vi "add_one_control_command.vi"(8 "error in":errorcluster, 9 "Controls Specs":T1[](array[typedef]), 10 "Instrument Command":string, 11 "VI Ref In":refnum<vi>) -> (0 "error out":errorcluster, 3 "VI Ref Out":refnum<vi>)   [LabVIEW 2018]
uses:
  TypeDefinitions/single_control_spec.ctl
  TypeDefinitions/control_data_type.ctl
  TypeDefinitions/control_class.ctl
  TypeDefinitions/ring_string_and_value.ctl
  Iternl/ConverttStr/TypeDefinitions/conver_strings_types.ctl
  Misc/AddNode/TypeDefinitions/node_types.ctl
  Iternl/CalPos/CmdToStr/TypeDefinitions/main_position_types.ctl
  Iternl/GetNodeTerm/StringProcessingNode/TypeDefinitions/string_node_type.ctl
  Iternl/ConttWire/TypeDefines/connect_with_last_node_types.ctl
  Iternl/AddObj/AddControl/TypeDefinitions/bd_control_type.ctl
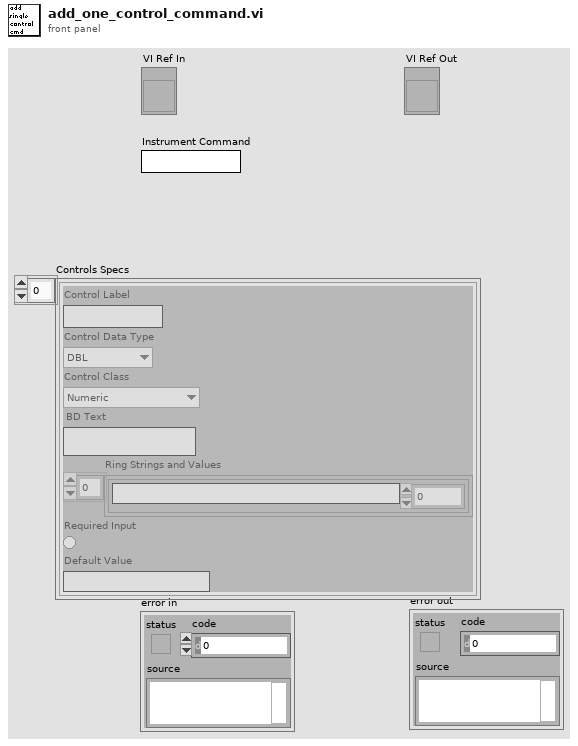
[diagram p1: front panel]
types:
  T1 = typedef "single_control_spec.ctl" = cluster{"Control Label":string, "Control Data Type":T2, "Control Class":T3, "BD Text":string, "Ring Strings and Values":T4[], "Required Input":bool, "Default Value":string}
  T2 = typedef "control_data_type.ctl" = enum16{"DBL", "I32", "Boolean", "String", "U16", "U32", "EXT", "SGL", "I16", "U8", "I8", "I64", "U64", "Waveform", "Reference", "Variant", "Cluster"}
  T3 = typedef "control_class.ctl" = enum16{"Numeric", "Vertical Slide Switch", "Text Ring", "String", "Array", "VISAName", "WaveformGraph", "Cluster"}
  T4 = typedef "ring_string_and_value.ctl" = cluster{"String":string, "Value":dbl}
  T5 = typedef "string_node_type.ctl" = enum16{"FormatIntoString", "PickLine", "AppendTrueFalse", "ConcatenateStrings"}
  T6 = typedef "main_position_types.ctl" = enum16{"Node", "FormatNodeForMultipleControls", "BoolConstant", "FormatConstant", "1stSubNodeX"}
  T7 = typedef "node_types.ctl" = enum16{"FormatIntoString", "PickLine", "AppendTrueFalse", "VISAWrite", "SubVI", "ConcatenateStrings", "VISARead", "ProperyNode", "ScanFromString", "SpreadSheetStringToArray"}
  T8 = typedef "conver_strings_types.ctl" = enum16{"BooleanCMD", "RingCMD"}
  T9 = typedef "bd_control_type.ctl" = enum16{"Numeric", "Ring", "Boolean", "String", "VisaIn", "VisaOut", "Error In", "Error Out", "Array", "Waveform"}
  T10 = typedef "connect_with_last_node_types.ctl" = u16
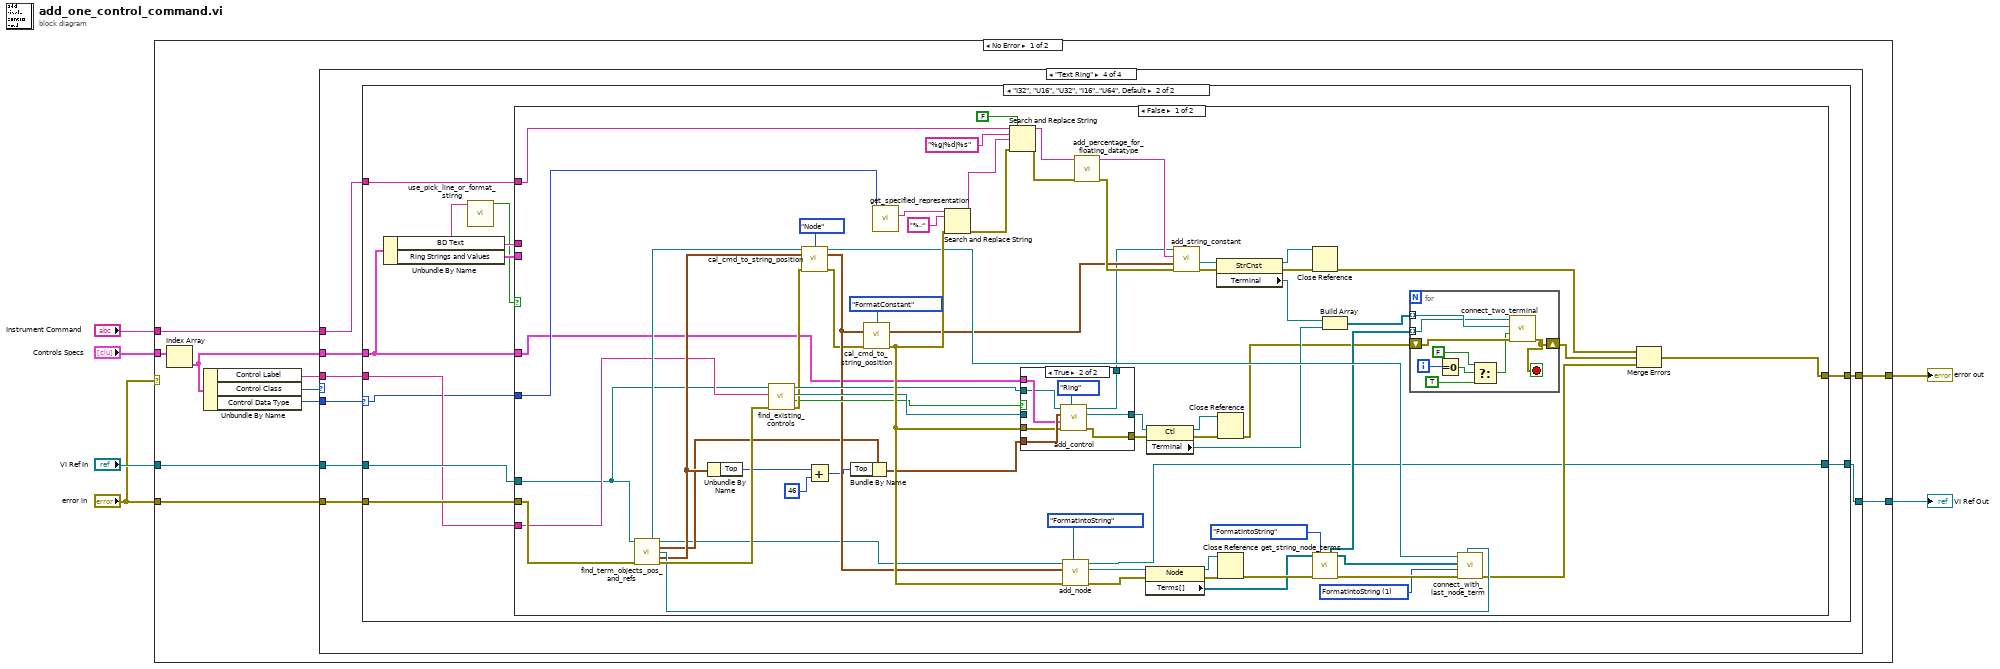
[diagram p0: block diagram]
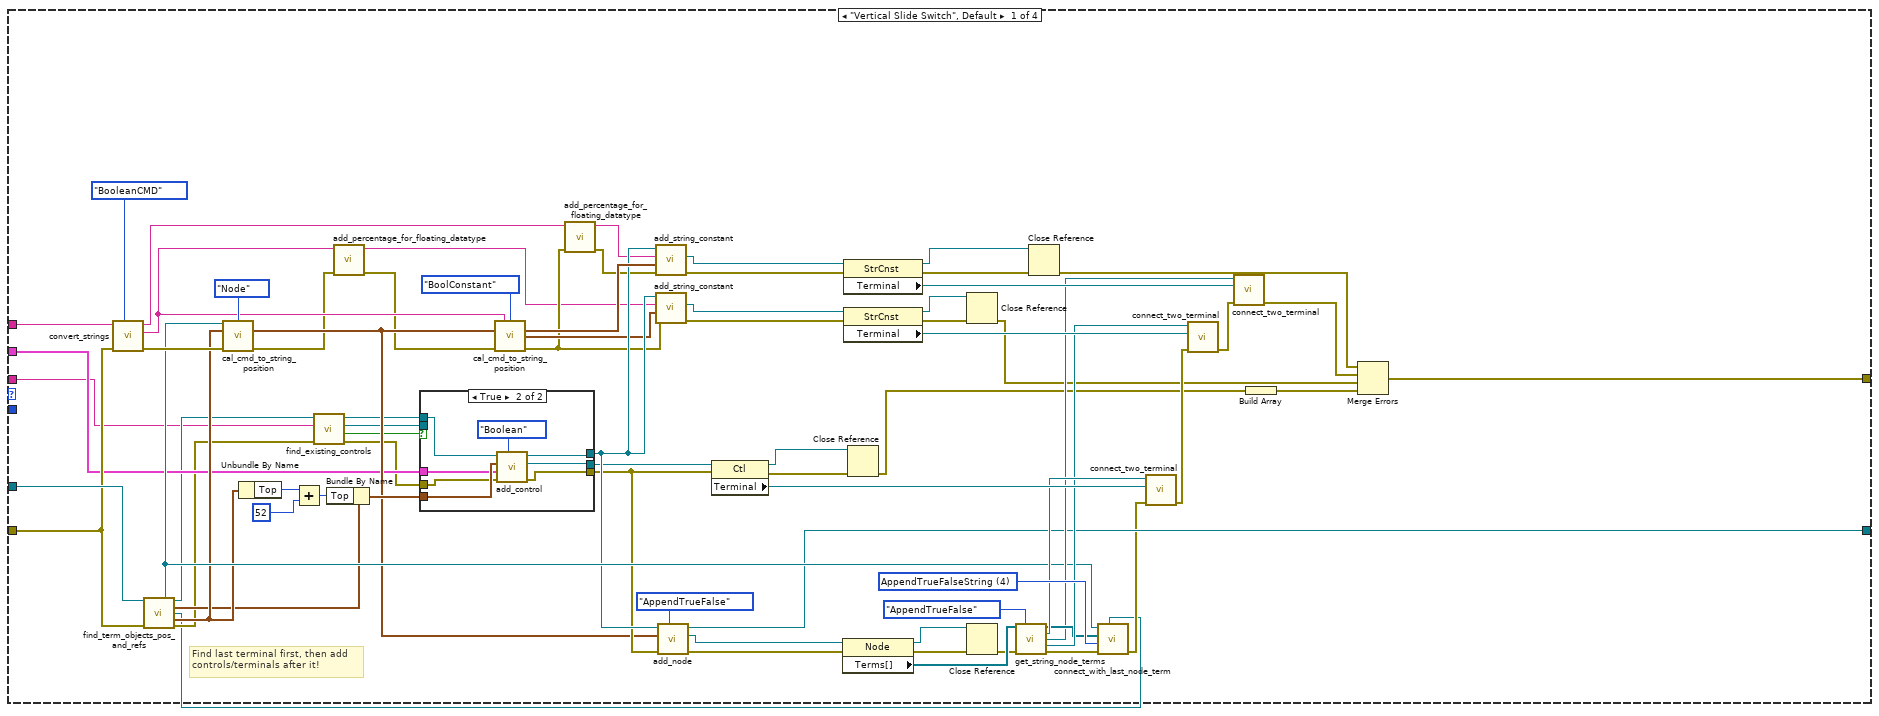
[diagram p2: hidden frame]
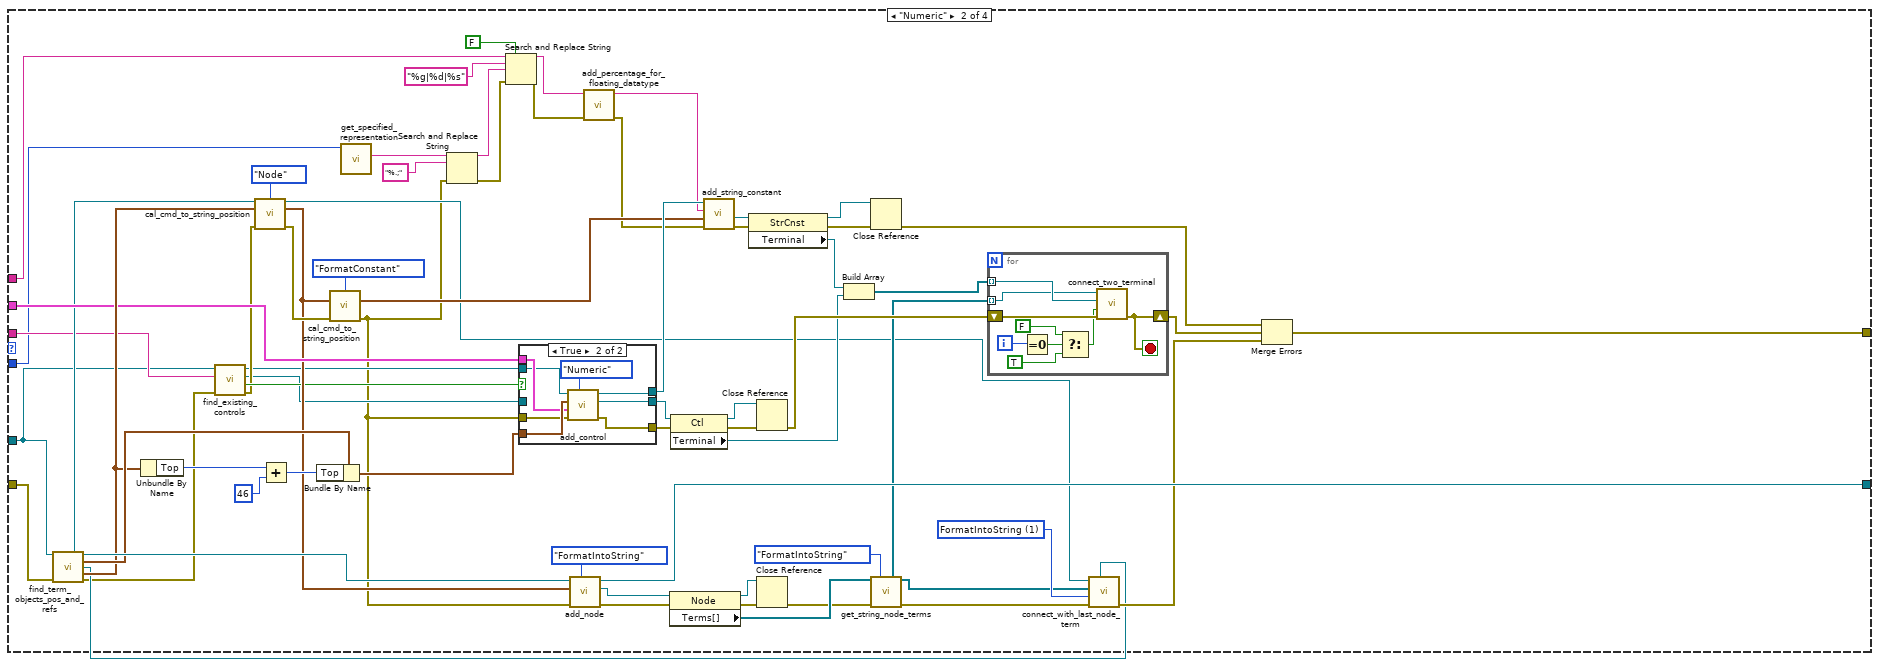
[diagram p4: hidden frame]
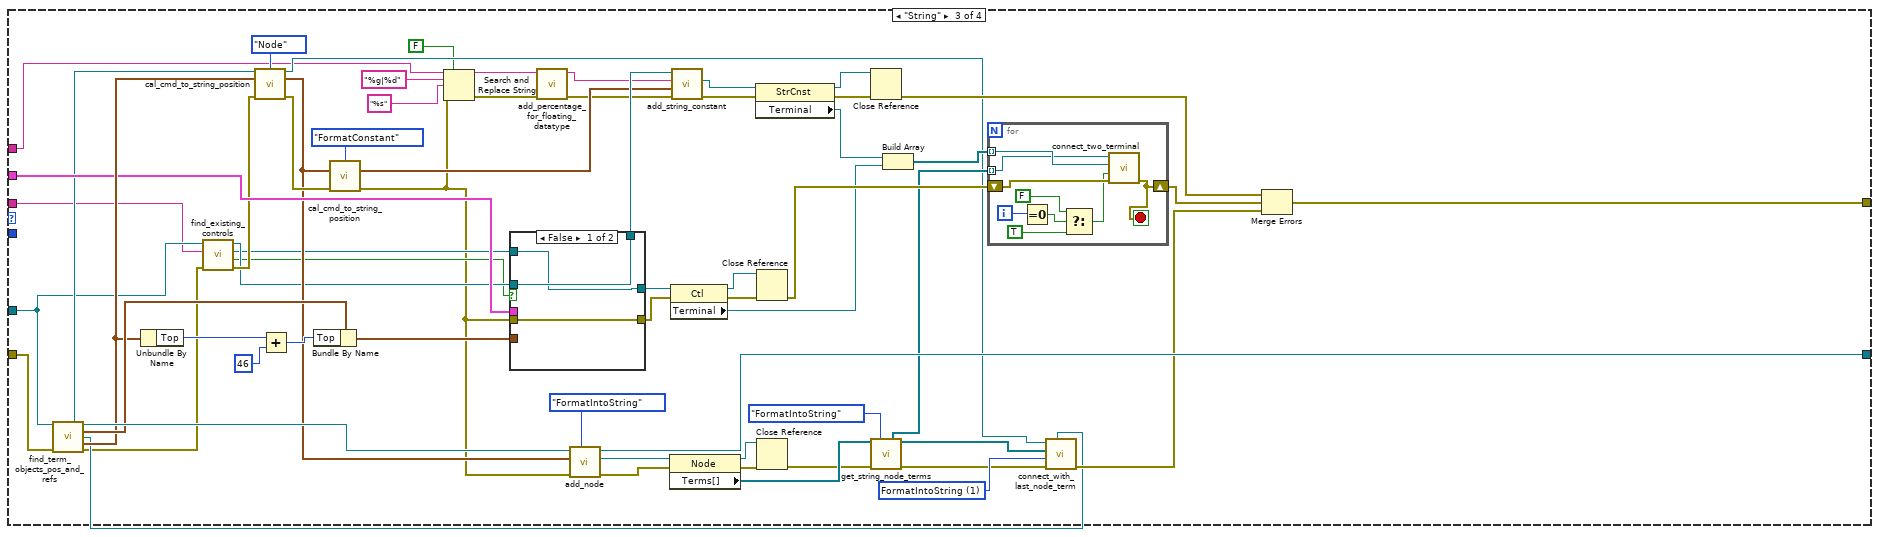
[diagram p6: hidden frame]
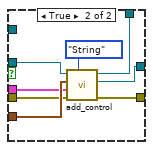
[diagram p7: hidden frame]
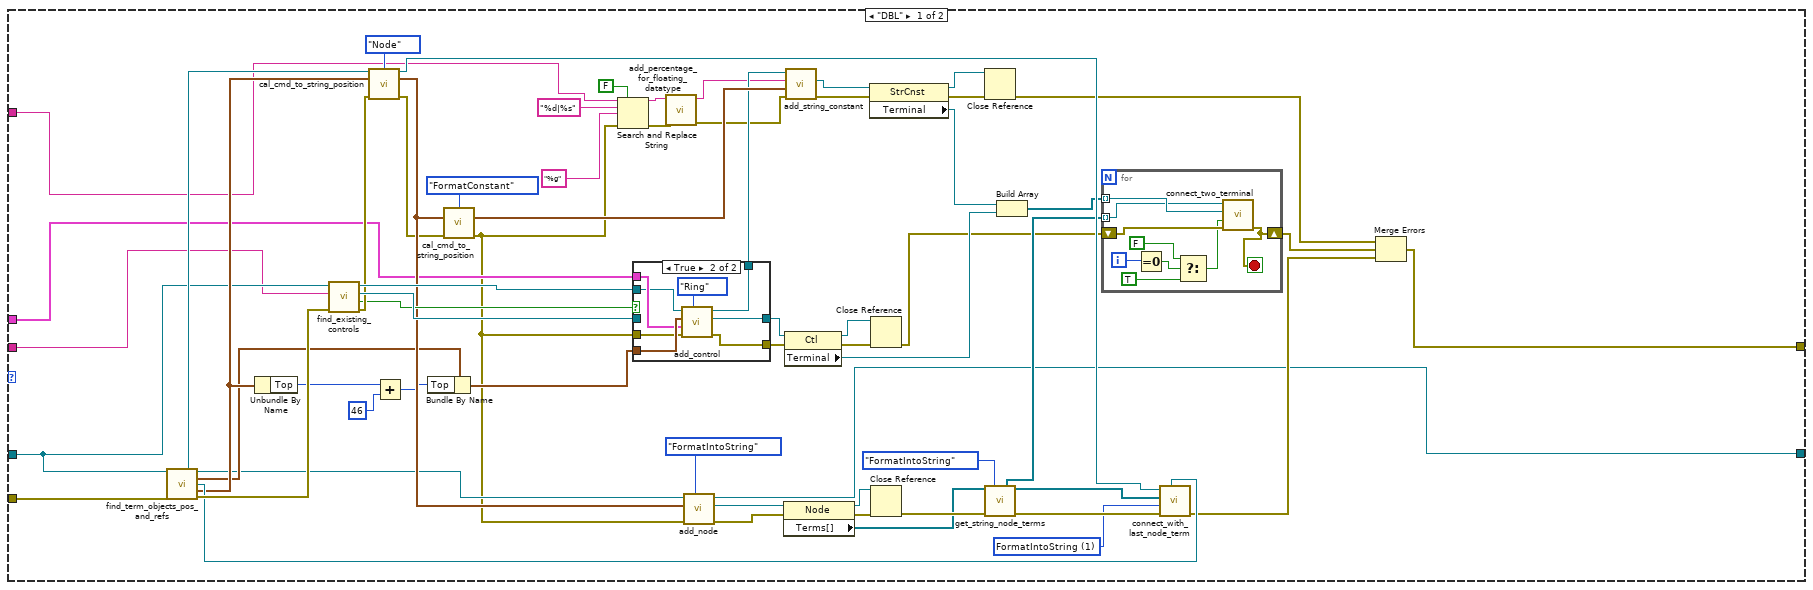
[diagram p8: hidden frame]
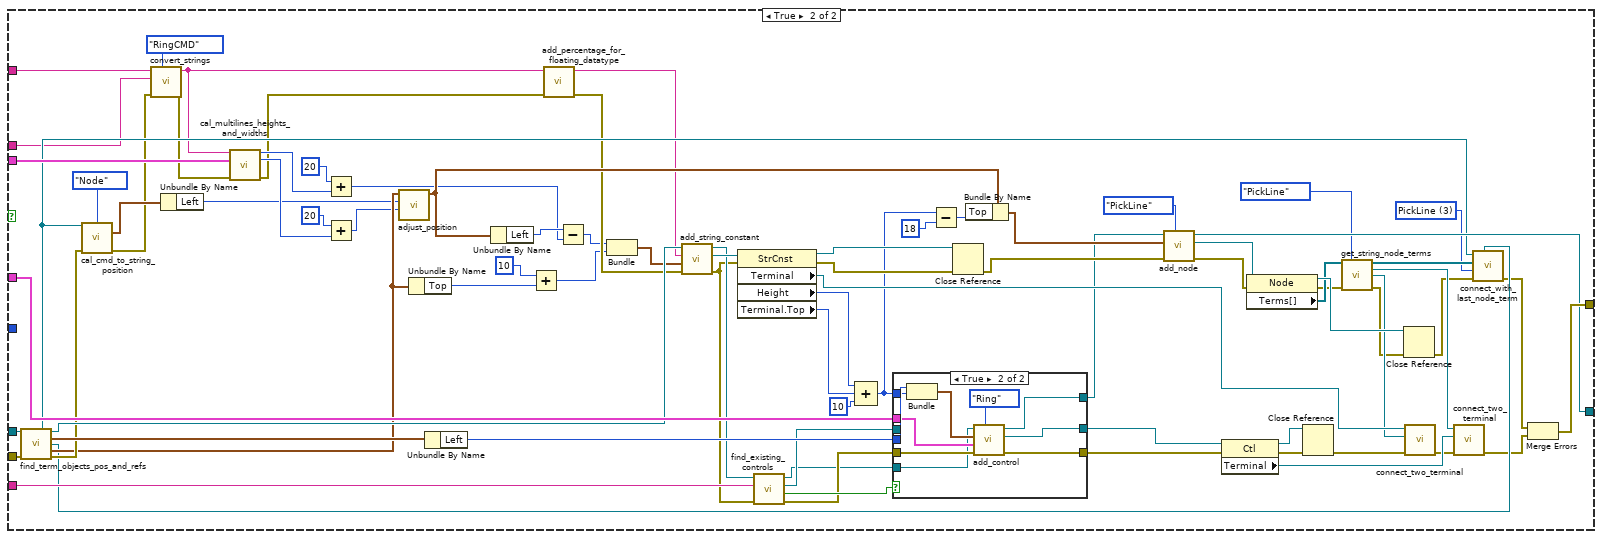
[diagram p11: hidden frame]
diagram:
  n1 = case shown="No Error" "error in" {
    selector: "error in" -> [_ w555]
    tunnel: "error in" -> [w15 _]
    tunnel: [w14 w555] -> w6
    tunnel: "Instrument Command" -> [w13 _]
    tunnel: [w11 w554] -> w4
    tunnel: "VI Ref In" -> [w10 w554]
    tunnel: "Controls Specs" -> [w9 _]
    frame No Error {
      n2 = Index Array(array=w9) -> (element=w16:T1)  [unwired: 1 in]
      n3 = Unbundle By Name(w16) -> ("Control Label"=w8:string, "Control Class"=w12:T3, "Control Data Type"=w7:T2)
      n4 = case shown="\"Text Ring\"" w12 {
        tunnel: w10 -> [w56 w120 w204 w277]
        tunnel: [w52 w154 w237 w275] -> w11
        tunnel: w16 -> [w48 w131 w214 w274]
        tunnel: w13 -> [w90 w113 w197 w279]
        tunnel: [w89 w139 w222 w276] -> w14
        tunnel: w15 -> [w55 w138 w221 w278]
        tunnel: w8 -> [w28 w121 w201 w273]
        tunnel: w7 -> [_ w112 _ w272]
        frame "Vertical Slide Switch", Default {
          w88 = T10 4 items=["AppendTrueFalseString"=4, "PickLine"=3, "FormatIntoString"=1] ("Terminal Index")
          # "Find last terminal first, then add \ncontrols/terminals after it!"
          n5 = call "convert_strings.vi"("Enum"=conver_strings_types."BooleanCMD", "error in (no error)"=w55, "Instrument Command"=w90) -> ("error out"=w86:errorcluster, "Disable String"=w21:string, "Ring CMD/Enable String"=w25:string)  [unwired: 1 in, 5 out]
          n6 = call "find_term_objects_pos_and_refs.vi"("VI Ref In"=w56, "error in (no error)"=w55) -> ("Last Function"=w63:refnum<vi>, "VI Ref Out"=w32:refnum<vi>, "Last Control Position"=w59:cluster{"Left":i32, "Top":i32}, "Last StrCnst Refnum"=w17:refnum<vi>, "Last Function Position"=w60:cluster{"Left":i32, "Top":i32}, "error out"=w31:errorcluster)  [unwired: 8 out]
          n7 = call "cal_cmd_to_string_position.vi"("Last Function Ref In"=w63, "Enum"=main_position_types."Node", "Main Node BD Position"=w60, "error in (no error)"=w86) -> ("Main Node Position/Enable Constant Position"=w49:cluster{"Left":u32, "Top":i32}, "error out"=w20:errorcluster)  [unwired: 3 in, 7 out]
          n8 = Unbundle By Name(w60) -> ("Top"=w58:i32)
          n9 = Add(x=w58, y=52) -> (x+y=w61:i32)
          n10 = call "find_existing_controls.vi"("error in (no error)"=w31, "Label Text"=w28, "VI Ref In"=w32) -> ("error out"=w30:errorcluster, "New Ctrl"=w26:bool, "Ctrl Ref Out"=w27:refnum<vi>, "VI Ref Out"=w29:refnum<vi>)  [unwired: 5 out]
          n11 = Bundle By Name(cluster=w59, "Top"=w61) -> (w57:cluster{"Left":i32, "Top":i32})
          n12 = call "add_percentage_for_floating_datatype.vi"("error in (no error)"=w20, "String In"=w21) -> ("error out"=w19:errorcluster, "String Out"=w18:string)  [unwired: 8 out]
          n13 = case shown="True" w26 {
            tunnel: w57 -> [_ w101]
            tunnel: [w93 w100] -> w54
            tunnel: [w91 w99] -> w50
            tunnel: w48 -> [_ w98]
            tunnel: [w92 w97] -> w44
            tunnel: w30 -> [w91 w95]
            tunnel: w29 -> [w93 w94]
            tunnel: w27 -> [w92 _]
            frame False {
            }
            frame True {
              n14 = call "add_control.vi"("Add Control Type"=bd_control_type."Boolean" ("Enum"), "error in (no error)"=w95, "Single Control Spec"=w98, "BD Position"=w101, "VI Ref In"=w94) -> ("error out"=w99:errorcluster, "Control Ref Out"=w97:refnum<vi>, "VI Ref Out"=w100:refnum<vi>)  [unwired: 4 out]
            }
          }
          n15 = call "cal_cmd_to_string_position.vi"("Disable String"=w21, "Enum"=main_position_types."BoolConstant", "Main Node BD Position"=w49, "error in (no error)"=w19) -> ("Main Node Position/Enable Constant Position"=w87:cluster{"Left":u32, "Top":i32}, "Disable Constant Position"=w36:cluster{u32, i32}, "error out"=w23:errorcluster)  [unwired: 3 in, 6 out]
          n16 = call "add_percentage_for_floating_datatype.vi"("error in (no error)"=w23, "String In"=w25) -> ("error out"=w22:errorcluster, "String Out"=w24:string)  [unwired: 8 out]
          n17 = call "add_string_constant.vi"("error in"=w22, "BD Position"=w87, "StringConstantValue"=w24, "VI Ref In"=w54) -> ("error out"=w84:errorcluster, "StrCnst Refnum"=w83:refnum<vi>)  [unwired: 6 out]
          n18 = call "add_string_constant.vi"("error in"=w23, "BD Position"=w36, "StringConstantValue"=w18, "VI Ref In"=w54) -> ("error out"=w85:errorcluster, "StrCnst Refnum"=w82:refnum<vi>)  [unwired: 6 out]
          n19 = call "add_node.vi"("Node Type"=node_types."AppendTrueFalse", "error in (no error)"=w50, "BD Position"=w49, "VI Ref In"=w54) -> ("error out"=w51:errorcluster, "Node Refnum"=w53:refnum<vi>, "VI Ref Out"=w52:refnum<vi>)  [unwired: 2 in, 3 out]
          n20 = property class="Ctl"(reference=w44, error in=w50) -> (reference out=w75:refnum<vi>, error out=w74:errorcluster, "Terminal"=w81:refnum<vi>)
          n21 = property class="Node"(reference=w53, error in=w51) -> (reference out=w73:refnum<vi>, error out=w72:errorcluster, "Terms[]"=w80:refnum<vi>[])
          n22 = property class="StrCnst"(reference=w83, error in=w84) -> (reference out=w70:refnum<vi>, error out=w69:errorcluster, "Terminal"=w79:refnum<vi>)
          n23 = property class="StrCnst"(reference=w82, error in=w85) -> (reference out=w68:refnum<vi>, error out=w67:errorcluster, "Terminal"=w78:refnum<vi>)
          n24 = Close Reference(reference=w75, error in (no error)=w74) -> (error out=w40:errorcluster)
          n25 = Close Reference(reference=w68, error in (no error)=w67) -> (error out=w41:errorcluster)
          n26 = Close Reference(reference=w73, error in (no error)=w72) -> (error out=w71:errorcluster)
          n27 = call "get_string_node_terms.vi"("Terms[] In"=w80, "Node Type"=string_node_type."AppendTrueFalse", "error in (no error)"=w71) -> ("Terms[]  Out"=w66:refnum<vi>[], "Pick Term"=w77:refnum<vi>, "Multiline Term/Enable Term/Concantenate Term"=w65:refnum<vi>, "Pick Line Output Term/Disable Term"=w76:refnum<vi>, "error out"=w64:errorcluster)  [unwired: 1 in, 7 out]
          n28 = Close Reference(reference=w70, error in (no error)=w69) -> (error out=w46:errorcluster)
          n29 = call "connect_with_last_node_term.vi"("Last StrCnst Refnum"=w17, "error in (no error)"=w64, "Terminal Index"=w88, "Terminals[]"=w66, "Last Function Ref In"=w63) -> ("error out"=w43:errorcluster)  [unwired: 6 out]
          n30 = call "connect_two_terminal.vi"("error in"=w43, "Terminal 2"=w81, "Terminal 1"=w77) -> ("error out"=w42:errorcluster)  [unwired: 1 in, 7 out]
          n31 = call "connect_two_terminal.vi"("error in"=w42, "Terminal 2"=w78, "Terminal 1"=w76) -> ("error out"=w47:errorcluster)  [unwired: 1 in, 7 out]
          n32 = call "connect_two_terminal.vi"("error in"=w47, "Terminal 2"=w79, "Terminal 1"=w65) -> ("error out"=w45:errorcluster)  [unwired: 1 in, 7 out]
          n33 = Build Array(w40) -> (w39:errorcluster[])
          n34 = Merge Errors(w46, w45, w41, w39) -> (w89:errorcluster)
        }
        frame "Numeric" {
          w168 = T10 1 items=["AppendTrueFalseString"=4, "PickLine"=3, "FormatIntoString"=1] ("Terminal Index")
          n35 = call "find_term_objects_pos_and_refs.vi"("VI Ref In"=w120, "error in (no error)"=w138) -> ("Last Function"=w127:refnum<vi>, "VI Ref Out"=w149:refnum<vi>, "Last Control Position"=w136:cluster{"Left":i32, "Top":i32}, "Last StrCnst Refnum"=w122:refnum<vi>, "Last Function Position"=w133:cluster{"Left":i32, "Top":i32}, "error out"=w119:errorcluster)  [unwired: 8 out]
          n36 = Unbundle By Name(w133) -> ("Top"=w132:i32)
          n37 = call "find_existing_controls.vi"("error in (no error)"=w119, "Label Text"=w121, "VI Ref In"=w120) -> ("error out"=w117:errorcluster, "New Ctrl"=w118:bool, "Ctrl Ref Out"=w115:refnum<vi>, "VI Ref Out"=w116:refnum<vi>)  [unwired: 5 out]
          n38 = call "cal_cmd_to_string_position.vi"("Last Function Ref In"=w127, "Enum"=main_position_types."Node", "Main Node BD Position"=w133, "error in (no error)"=w117) -> ("Last Function Ref Out"=w126:refnum<vi>, "Main Node Position/Enable Constant Position"=w129:cluster{"Left":u32, "Top":i32}, "error out"=w167:errorcluster)  [unwired: 3 in, 6 out]
          n39 = Add(x=w132, y=46) -> (x+y=w134:i32)
          n40 = Bundle By Name(cluster=w136, "Top"=w134) -> (w135:cluster{"Left":i32, "Top":i32})
          n41 = call "cal_cmd_to_string_position.vi"("Enum"=main_position_types."FormatConstant", "Main Node BD Position"=w129, "error in (no error)"=w167) -> ("Main Node Position/Enable Constant Position"=w128:cluster{"Left":u32, "Top":i32}, "error out"=w107:errorcluster)  [unwired: 4 in, 7 out]
          n42 = call "get_specified_representation.vi"("Control Data Type"=w112) -> ("Format String"=w110:string)  [unwired: 10 out]
          n43 = Search and Replace String(input string=w110, search string="%.;", error in=w107) -> (result string=w108:string, error out=w106:errorcluster)  [unwired: 7 out]
          n44 = Search and Replace String(replace all?=FALSE ("replace all? (F)"), input string=w113, search string="%g|%d|%s", replace string=w108, error in=w106) -> (result string=w104:string, error out=w103:errorcluster)  [unwired: 5 out]
          n45 = case shown="True" w118 {
            tunnel: [w170 w179] -> w151
            tunnel: [w171 w178] -> w150
            tunnel: [w169 w177] -> w148
            tunnel: w135 -> [_ w176]
            tunnel: w107 -> [w169 w175]
            tunnel: w131 -> [_ w174]
            tunnel: w116 -> [w171 w172]
            tunnel: w115 -> [w170 _]
            frame False {
            }
            frame True {
              n46 = call "add_control.vi"("Add Control Type"=bd_control_type."Numeric" ("Enum"), "error in (no error)"=w175, "Single Control Spec"=w174, "BD Position"=w176, "VI Ref In"=w172) -> ("error out"=w177:errorcluster, "Control Ref Out"=w179:refnum<vi>, "VI Ref Out"=w178:refnum<vi>)  [unwired: 4 out]
            }
          }
          n47 = call "add_node.vi"("Node Type"=node_types."FormatIntoString", "error in (no error)"=w107, "BD Position"=w129, "VI Ref In"=w149) -> ("error out"=w165:errorcluster, "Node Refnum"=w140:refnum<vi>, "VI Ref Out"=w154:refnum<vi>)  [unwired: 2 in, 3 out]
          n48 = call "add_percentage_for_floating_datatype.vi"("error in (no error)"=w103, "String In"=w104) -> ("error out"=w102:errorcluster, "String Out"=w105:string)  [unwired: 8 out]
          n49 = property class="Node"(reference=w140, error in=w165) -> (reference out=w160:refnum<vi>, error out=w159:errorcluster, "Terms[]"=w163:refnum<vi>[])
          n50 = property class="Ctl"(reference=w151, error in=w148) -> (reference out=w162:refnum<vi>, error out=w161:errorcluster, "Terminal"=w144:refnum<vi>)
          n51 = call "add_string_constant.vi"("error in"=w102, "BD Position"=w128, "StringConstantValue"=w105, "VI Ref In"=w150) -> ("error out"=w166:errorcluster, "StrCnst Refnum"=w164:refnum<vi>)  [unwired: 6 out]
          n52 = property class="StrCnst"(reference=w164, error in=w166) -> (reference out=w157:refnum<vi>, error out=w156:errorcluster, "Terminal"=w145:refnum<vi>)
          n53 = Close Reference(reference=w162, error in (no error)=w161) -> (error out=w152:errorcluster)
          n54 = Close Reference(reference=w160, error in (no error)=w159) -> (error out=w158:errorcluster)
          n55 = Build Array(w145, w144) -> (w143:refnum<vi>[])
          n56 = Close Reference(reference=w157, error in (no error)=w156) -> (error out=w141:errorcluster)
          n57 = call "get_string_node_terms.vi"("Terms[] In"=w163, "Node Type"=string_node_type."FormatIntoString", "error in (no error)"=w158) -> ("Format Terms Out"=w142:refnum<vi>[], "Terms[]  Out"=w155:refnum<vi>[], "error out"=w153:errorcluster)  [unwired: 1 in, 9 out]
          n58 = for {
            shift-right: [w180] -> w147
            shift-left: w152 -> [w188]
            tunnel: w143 -> [w187] mode=indexing
            tunnel: w142 -> [w186] mode=indexing
            i -> [w185]
            stop <- w180 stop-if-true
            n59 = Equal To 0?(x=w185) -> (x = 0?=w184:bool)
            n60 = Select(t=FALSE ("Auto Route? (T)"), s=w184, f=TRUE ("Auto Route? (T)")) -> (s? t:f=w181:bool)
            n61 = call "connect_two_terminal.vi"("error in"=w188, "Auto Route? (T)"=w181, "Terminal 2"=w187, "Terminal 1"=w186) -> ("error out"=w180:errorcluster)  [unwired: 7 out]
          }
          n62 = call "connect_with_last_node_term.vi"("Last StrCnst Refnum"=w122, "error in (no error)"=w153, "Terminal Index"=w168, "Terminals[]"=w155, "Last Function Ref In"=w126) -> ("error out"=w146:errorcluster)  [unwired: 6 out]
          n63 = Merge Errors(w141, w147, w146) -> (w139:errorcluster)
        }
        frame "String" {
          w251 = T10 1 items=["AppendTrueFalseString"=4, "PickLine"=3, "FormatIntoString"=1] ("Terminal Index")
          n64 = call "find_term_objects_pos_and_refs.vi"("VI Ref In"=w204, "error in (no error)"=w221) -> ("Last Function"=w210:refnum<vi>, "VI Ref Out"=w232:refnum<vi>, "Last Control Position"=w219:cluster{"Left":i32, "Top":i32}, "Last StrCnst Refnum"=w205:refnum<vi>, "Last Function Position"=w216:cluster{"Left":i32, "Top":i32}, "error out"=w203:errorcluster)  [unwired: 8 out]
          n65 = Unbundle By Name(w216) -> ("Top"=w215:i32)
          n66 = call "find_existing_controls.vi"("error in (no error)"=w203, "Label Text"=w201, "VI Ref In"=w204) -> ("error out"=w202:errorcluster, "New Ctrl"=w199:bool, "Ctrl Ref Out"=w198:refnum<vi>, "VI Ref Out"=w200:refnum<vi>)  [unwired: 5 out]
          n67 = call "cal_cmd_to_string_position.vi"("Last Function Ref In"=w210, "Enum"=main_position_types."Node", "Main Node BD Position"=w216, "error in (no error)"=w202) -> ("Last Function Ref Out"=w209:refnum<vi>, "Main Node Position/Enable Constant Position"=w212:cluster{"Left":u32, "Top":i32}, "error out"=w250:errorcluster)  [unwired: 3 in, 6 out]
          n68 = Add(x=w215, y=46) -> (x+y=w217:i32)
          n69 = Bundle By Name(cluster=w219, "Top"=w217) -> (w218:cluster{"Left":i32, "Top":i32})
          n70 = call "cal_cmd_to_string_position.vi"("Enum"=main_position_types."FormatConstant", "Main Node BD Position"=w212, "error in (no error)"=w250) -> ("Main Node Position/Enable Constant Position"=w211:cluster{"Left":u32, "Top":i32}, "error out"=w194:errorcluster)  [unwired: 4 in, 7 out]
          n71 = Search and Replace String(replace all?=FALSE ("replace all? (F)"), input string=w197, search string="%g|%d", replace string="%s" ("replace string (\"\")"), error in=w194) -> (result string=w192:string, error out=w190:errorcluster)  [unwired: 5 out]
          n72 = case shown="False" w199 {
            tunnel: [w253 w262] -> w234
            tunnel: [w254 w261] -> w233
            tunnel: [w252 w260] -> w231
            tunnel: w218 -> [_ w259]
            tunnel: w194 -> [w252 w258]
            tunnel: w214 -> [_ w257]
            tunnel: w200 -> [w254 w255]
            tunnel: w198 -> [w253 _]
            frame False {
            }
            frame True {
              n73 = call "add_control.vi"("Add Control Type"=bd_control_type."String" ("Enum"), "error in (no error)"=w258, "Single Control Spec"=w257, "BD Position"=w259, "VI Ref In"=w255) -> ("error out"=w260:errorcluster, "Control Ref Out"=w262:refnum<vi>, "VI Ref Out"=w261:refnum<vi>)  [unwired: 4 out]
            }
          }
          n74 = call "add_percentage_for_floating_datatype.vi"("error in (no error)"=w190, "String In"=w192) -> ("error out"=w189:errorcluster, "String Out"=w191:string)  [unwired: 8 out]
          n75 = call "add_node.vi"("Node Type"=node_types."FormatIntoString", "error in (no error)"=w194, "BD Position"=w212, "VI Ref In"=w232) -> ("error out"=w248:errorcluster, "Node Refnum"=w223:refnum<vi>, "VI Ref Out"=w237:refnum<vi>)  [unwired: 2 in, 3 out]
          n76 = property class="Node"(reference=w223, error in=w248) -> (reference out=w243:refnum<vi>, error out=w242:errorcluster, "Terms[]"=w246:refnum<vi>[])
          n77 = property class="Ctl"(reference=w234, error in=w231) -> (reference out=w245:refnum<vi>, error out=w244:errorcluster, "Terminal"=w227:refnum<vi>)
          n78 = call "add_string_constant.vi"("error in"=w189, "BD Position"=w211, "StringConstantValue"=w191, "VI Ref In"=w233) -> ("error out"=w249:errorcluster, "StrCnst Refnum"=w247:refnum<vi>)  [unwired: 6 out]
          n79 = property class="StrCnst"(reference=w247, error in=w249) -> (reference out=w240:refnum<vi>, error out=w239:errorcluster, "Terminal"=w228:refnum<vi>)
          n80 = Close Reference(reference=w245, error in (no error)=w244) -> (error out=w235:errorcluster)
          n81 = Close Reference(reference=w243, error in (no error)=w242) -> (error out=w241:errorcluster)
          n82 = Close Reference(reference=w240, error in (no error)=w239) -> (error out=w224:errorcluster)
          n83 = call "get_string_node_terms.vi"("Terms[] In"=w246, "Node Type"=string_node_type."FormatIntoString", "error in (no error)"=w241) -> ("Format Terms Out"=w225:refnum<vi>[], "Terms[]  Out"=w238:refnum<vi>[], "error out"=w236:errorcluster)  [unwired: 1 in, 9 out]
          n84 = Build Array(w228, w227) -> (w226:refnum<vi>[])
          n85 = for {
            shift-right: [w263] -> w230
            shift-left: w235 -> [w271]
            tunnel: w226 -> [w270] mode=indexing
            tunnel: w225 -> [w269] mode=indexing
            i -> [w268]
            stop <- w263 stop-if-true
            n86 = Equal To 0?(x=w268) -> (x = 0?=w267:bool)
            n87 = Select(t=FALSE ("Auto Route? (T)"), s=w267, f=TRUE ("Auto Route? (T)")) -> (s? t:f=w264:bool)
            n88 = call "connect_two_terminal.vi"("error in"=w271, "Auto Route? (T)"=w264, "Terminal 2"=w270, "Terminal 1"=w269) -> ("error out"=w263:errorcluster)  [unwired: 7 out]
          }
          n89 = call "connect_with_last_node_term.vi"("Last StrCnst Refnum"=w205, "error in (no error)"=w236, "Terminal Index"=w251, "Terminals[]"=w238, "Last Function Ref In"=w209) -> ("error out"=w229:errorcluster)  [unwired: 6 out]
          n90 = Merge Errors(w224, w230, w229) -> (w222:errorcluster)
        }
        frame "Text Ring" {
          n91 = case shown="\"I32\", \"U16\", \"U32\", \"I16\"..\"U64\", Default" w272 {
            selector: w272 -> [_ w363]
            tunnel: w279 -> [w286 w373]
            tunnel: w278 -> [w294 w372]
            tunnel: w277 -> [w293 w371]
            tunnel: [w290 w370] -> w276
            tunnel: [w289 w369] -> w275
            tunnel: w274 -> [w292 w368]
            tunnel: w273 -> [w291 w367]
            frame "DBL" {
              w295 = T10 1 items=["AppendTrueFalseString"=4, "PickLine"=3, "FormatIntoString"=1] ("Terminal Index")
              n92 = call "find_term_objects_pos_and_refs.vi"("VI Ref In"=w293, "error in (no error)"=w294) -> ("Last Function"=w332:refnum<vi>, "VI Ref Out"=w313:refnum<vi>, "Last Control Position"=w324:cluster{"Left":i32, "Top":i32}, "Last StrCnst Refnum"=w337:refnum<vi>, "Last Function Position"=w327:cluster{"Left":i32, "Top":i32}, "error out"=w338:errorcluster)  [unwired: 8 out]
              n93 = Unbundle By Name(w327) -> ("Top"=w328:i32)
              n94 = call "find_existing_controls.vi"("error in (no error)"=w338, "Label Text"=w291, "VI Ref In"=w293) -> ("error out"=w340:errorcluster, "New Ctrl"=w339:bool, "Ctrl Ref Out"=w342:refnum<vi>, "VI Ref Out"=w341:refnum<vi>)  [unwired: 5 out]
              n95 = call "cal_cmd_to_string_position.vi"("Last Function Ref In"=w332, "Enum"=main_position_types."Node", "Main Node BD Position"=w327, "error in (no error)"=w340) -> ("Last Function Ref Out"=w333:refnum<vi>, "Main Node Position/Enable Constant Position"=w330:cluster{"Left":u32, "Top":i32}, "error out"=w296:errorcluster)  [unwired: 3 in, 6 out]
              n96 = Add(x=w328, y=46) -> (x+y=w326:i32)
              n97 = Bundle By Name(cluster=w324, "Top"=w326) -> (w325:cluster{"Left":i32, "Top":i32})
              n98 = call "cal_cmd_to_string_position.vi"("Enum"=main_position_types."FormatConstant", "Main Node BD Position"=w330, "error in (no error)"=w296) -> ("Main Node Position/Enable Constant Position"=w331:cluster{"Left":u32, "Top":i32}, "error out"=w281:errorcluster)  [unwired: 4 in, 7 out]
              n99 = Search and Replace String(replace all?=FALSE ("replace all? (F)"), input string=w286, search string="%d|%s", replace string="%g" ("replace string (\"\")"), error in=w281) -> (result string=w284:string, error out=w282:errorcluster)  [unwired: 5 out]
              n100 = case shown="True" w339 {
                tunnel: [w344 w353] -> w311
                tunnel: [w345 w352] -> w312
                tunnel: [w343 w351] -> w314
                tunnel: w325 -> [_ w350]
                tunnel: w281 -> [w343 w349]
                tunnel: w292 -> [_ w348]
                tunnel: w341 -> [w345 w346]
                tunnel: w342 -> [w344 _]
                frame False {
                }
                frame True {
                  n101 = call "add_control.vi"("Add Control Type"=bd_control_type."Ring" ("Enum"), "error in (no error)"=w349, "Single Control Spec"=w348, "BD Position"=w350, "VI Ref In"=w346) -> ("error out"=w351:errorcluster, "Control Ref Out"=w353:refnum<vi>, "VI Ref Out"=w352:refnum<vi>)  [unwired: 4 out]
                }
              }
              n102 = call "add_percentage_for_floating_datatype.vi"("error in (no error)"=w282, "String In"=w284) -> ("error out"=w280:errorcluster, "String Out"=w283:string)  [unwired: 8 out]
              n103 = call "add_node.vi"("Node Type"=node_types."FormatIntoString", "error in (no error)"=w281, "BD Position"=w330, "VI Ref In"=w313) -> ("error out"=w298:errorcluster, "Node Refnum"=w322:refnum<vi>, "VI Ref Out"=w289:refnum<vi>)  [unwired: 2 in, 3 out]
              n104 = property class="Node"(reference=w322, error in=w298) -> (reference out=w303:refnum<vi>, error out=w304:errorcluster, "Terms[]"=w300:refnum<vi>[])
              n105 = property class="Ctl"(reference=w311, error in=w314) -> (reference out=w301:refnum<vi>, error out=w302:errorcluster, "Terminal"=w318:refnum<vi>)
              n106 = call "add_string_constant.vi"("error in"=w280, "BD Position"=w331, "StringConstantValue"=w283, "VI Ref In"=w312) -> ("error out"=w297:errorcluster, "StrCnst Refnum"=w299:refnum<vi>)  [unwired: 6 out]
              n107 = property class="StrCnst"(reference=w299, error in=w297) -> (reference out=w306:refnum<vi>, error out=w307:errorcluster, "Terminal"=w317:refnum<vi>)
              n108 = Close Reference(reference=w301, error in (no error)=w302) -> (error out=w310:errorcluster)
              n109 = Close Reference(reference=w303, error in (no error)=w304) -> (error out=w305:errorcluster)
              n110 = Close Reference(reference=w306, error in (no error)=w307) -> (error out=w321:errorcluster)
              n111 = call "get_string_node_terms.vi"("Terms[] In"=w300, "Node Type"=string_node_type."FormatIntoString", "error in (no error)"=w305) -> ("Format Terms Out"=w320:refnum<vi>[], "Terms[]  Out"=w308:refnum<vi>[], "error out"=w309:errorcluster)  [unwired: 1 in, 9 out]
              n112 = Build Array(w317, w318) -> (w319:refnum<vi>[])
              n113 = for {
                shift-right: [w354] -> w315
                shift-left: w310 -> [w362]
                tunnel: w319 -> [w361] mode=indexing
                tunnel: w320 -> [w360] mode=indexing
                i -> [w359]
                stop <- w354 stop-if-true
                n114 = Equal To 0?(x=w359) -> (x = 0?=w358:bool)
                n115 = Select(t=FALSE ("Auto Route? (T)"), s=w358, f=TRUE ("Auto Route? (T)")) -> (s? t:f=w355:bool)
                n116 = call "connect_two_terminal.vi"("error in"=w362, "Auto Route? (T)"=w355, "Terminal 2"=w361, "Terminal 1"=w360) -> ("error out"=w354:errorcluster)  [unwired: 7 out]
              }
              n117 = call "connect_with_last_node_term.vi"("Last StrCnst Refnum"=w337, "error in (no error)"=w309, "Terminal Index"=w295, "Terminals[]"=w308, "Last Function Ref In"=w333) -> ("error out"=w316:errorcluster)  [unwired: 6 out]
              n118 = Merge Errors(w321, w315, w316) -> (w290:errorcluster)
            }
            frame "I32", "U16", "U32", "I16".."U64", Default {
              n119 = Unbundle By Name(w368) -> ("BD Text"=w365:string, "Ring Strings and Values"=w366:T4[])
              n120 = call "use_pick_line_or_format_stirng.vi"("BD"=w365) -> ("Pick Line Node?"=w364:bool)  [unwired: 10 out]
              n121 = case shown="False" w364 {
                tunnel: w373 -> [w380 w540]
                tunnel: w372 -> [w382 w539]
                tunnel: w371 -> [w377 w538]
                tunnel: [w375 w537] -> w370
                tunnel: [w376 w536] -> w369
                tunnel: w368 -> [w379 w535]
                tunnel: w367 -> [w378 w534]
                tunnel: w366 -> [_ w533]
                tunnel: w365 -> [_ w497]
                tunnel: w363 -> [w381 _]
                frame False {
                  w383 = T10 1 items=["AppendTrueFalseString"=4, "PickLine"=3, "FormatIntoString"=1] ("Terminal Index")
                  n122 = call "find_term_objects_pos_and_refs.vi"("VI Ref In"=w377, "error in (no error)"=w382) -> ("Last Function"=w420:refnum<vi>, "VI Ref Out"=w401:refnum<vi>, "Last Control Position"=w412:cluster{"Left":i32, "Top":i32}, "Last StrCnst Refnum"=w425:refnum<vi>, "Last Function Position"=w415:cluster{"Left":i32, "Top":i32}, "error out"=w426:errorcluster)  [unwired: 8 out]
                  n123 = Unbundle By Name(w415) -> ("Top"=w416:i32)
                  n124 = call "find_existing_controls.vi"("error in (no error)"=w426, "Label Text"=w378, "VI Ref In"=w377) -> ("error out"=w428:errorcluster, "New Ctrl"=w427:bool, "Ctrl Ref Out"=w430:refnum<vi>, "VI Ref Out"=w429:refnum<vi>)  [unwired: 5 out]
                  n125 = call "cal_cmd_to_string_position.vi"("Last Function Ref In"=w420, "Enum"=main_position_types."Node", "Main Node BD Position"=w415, "error in (no error)"=w428) -> ("Last Function Ref Out"=w421:refnum<vi>, "Main Node Position/Enable Constant Position"=w418:cluster{"Left":u32, "Top":i32}, "error out"=w384:errorcluster)  [unwired: 3 in, 6 out]
                  n126 = Add(x=w416, y=46) -> (x+y=w414:i32)
                  n127 = Bundle By Name(cluster=w412, "Top"=w414) -> (w413:cluster{"Left":i32, "Top":i32})
                  n128 = call "cal_cmd_to_string_position.vi"("Enum"=main_position_types."FormatConstant", "Main Node BD Position"=w418, "error in (no error)"=w384) -> ("Main Node Position/Enable Constant Position"=w419:cluster{"Left":u32, "Top":i32}, "error out"=w435:errorcluster)  [unwired: 4 in, 7 out]
                  n129 = call "get_specified_representation.vi"("Control Data Type"=w381) -> ("Format String"=w374:string)  [unwired: 10 out]
                  n130 = Search and Replace String(input string=w374, search string="%.;", error in=w435) -> (result string=w434:string, error out=w436:errorcluster)  [unwired: 7 out]
                  n131 = Search and Replace String(replace all?=FALSE ("replace all? (F)"), input string=w380, search string="%g|%d|%s", replace string=w434, error in=w436) -> (result string=w438:string, error out=w439:errorcluster)  [unwired: 5 out]
                  n132 = case shown="True" w427 {
                    tunnel: [w442 w451] -> w399
                    tunnel: [w443 w450] -> w400
                    tunnel: [w441 w449] -> w402
                    tunnel: w413 -> [_ w448]
                    tunnel: w435 -> [w441 w447]
                    tunnel: w379 -> [_ w446]
                    tunnel: w429 -> [w443 w444]
                    tunnel: w430 -> [w442 _]
                    frame False {
                    }
                    frame True {
                      n133 = call "add_control.vi"("Add Control Type"=bd_control_type."Ring" ("Enum"), "error in (no error)"=w447, "Single Control Spec"=w446, "BD Position"=w448, "VI Ref In"=w444) -> ("error out"=w449:errorcluster, "Control Ref Out"=w451:refnum<vi>, "VI Ref Out"=w450:refnum<vi>)  [unwired: 4 out]
                    }
                  }
                  n134 = call "add_node.vi"("Node Type"=node_types."FormatIntoString", "error in (no error)"=w435, "BD Position"=w418, "VI Ref In"=w401) -> ("error out"=w386:errorcluster, "Node Refnum"=w410:refnum<vi>, "VI Ref Out"=w376:refnum<vi>)  [unwired: 2 in, 3 out]
                  n135 = call "add_percentage_for_floating_datatype.vi"("error in (no error)"=w439, "String In"=w438) -> ("error out"=w440:errorcluster, "String Out"=w437:string)  [unwired: 8 out]
                  n136 = property class="Node"(reference=w410, error in=w386) -> (reference out=w391:refnum<vi>, error out=w392:errorcluster, "Terms[]"=w388:refnum<vi>[])
                  n137 = property class="Ctl"(reference=w399, error in=w402) -> (reference out=w389:refnum<vi>, error out=w390:errorcluster, "Terminal"=w406:refnum<vi>)
                  n138 = call "add_string_constant.vi"("error in"=w440, "BD Position"=w419, "StringConstantValue"=w437, "VI Ref In"=w400) -> ("error out"=w385:errorcluster, "StrCnst Refnum"=w387:refnum<vi>)  [unwired: 6 out]
                  n139 = property class="StrCnst"(reference=w387, error in=w385) -> (reference out=w394:refnum<vi>, error out=w395:errorcluster, "Terminal"=w405:refnum<vi>)
                  n140 = Close Reference(reference=w389, error in (no error)=w390) -> (error out=w398:errorcluster)
                  n141 = Close Reference(reference=w391, error in (no error)=w392) -> (error out=w393:errorcluster)
                  n142 = Close Reference(reference=w394, error in (no error)=w395) -> (error out=w409:errorcluster)
                  n143 = call "get_string_node_terms.vi"("Terms[] In"=w388, "Node Type"=string_node_type."FormatIntoString", "error in (no error)"=w393) -> ("Format Terms Out"=w408:refnum<vi>[], "Terms[]  Out"=w396:refnum<vi>[], "error out"=w397:errorcluster)  [unwired: 1 in, 9 out]
                  n144 = Build Array(w405, w406) -> (w407:refnum<vi>[])
                  n145 = for {
                    shift-right: [w452] -> w403
                    shift-left: w398 -> [w460]
                    tunnel: w407 -> [w459] mode=indexing
                    tunnel: w408 -> [w458] mode=indexing
                    i -> [w457]
                    stop <- w452 stop-if-true
                    n146 = Equal To 0?(x=w457) -> (x = 0?=w456:bool)
                    n147 = Select(t=FALSE ("Auto Route? (T)"), s=w456, f=TRUE ("Auto Route? (T)")) -> (s? t:f=w453:bool)
                    n148 = call "connect_two_terminal.vi"("error in"=w460, "Auto Route? (T)"=w453, "Terminal 2"=w459, "Terminal 1"=w458) -> ("error out"=w452:errorcluster)  [unwired: 7 out]
                  }
                  n149 = call "connect_with_last_node_term.vi"("Last StrCnst Refnum"=w425, "error in (no error)"=w397, "Terminal Index"=w383, "Terminals[]"=w396, "Last Function Ref In"=w421) -> ("error out"=w404:errorcluster)  [unwired: 6 out]
                  n150 = Merge Errors(w409, w403, w404) -> (w375:errorcluster)
                }
                frame True {
                  w488 = u16 3 items=["AppendTrueFalseString"=4, "PickLine"=3, "FormatIntoString"=1] ("Terminal Index")
                  n151 = call "find_term_objects_pos_and_refs.vi"("VI Ref In"=w538, "error in (no error)"=w539) -> ("Last Function"=w523:refnum<vi>, "VI Ref Out"=w532:refnum<vi>, "Last Control Position"=w528:cluster{"Left":i32, "Top":i32}, "Last StrCnst Refnum"=w507:refnum<vi>, "Last Function Position"=w513:cluster{"Left":i32, "Top":i32}, "error out"=w520:errorcluster)  [unwired: 8 out]
                  n152 = call "cal_cmd_to_string_position.vi"("Last Function Ref In"=w523, "Enum"=main_position_types."Node", "error in (no error)"=w520) -> ("Main Node Position/Enable Constant Position"=w521:cluster{"Left":u32, "Top":i32}, "error out"=w515:errorcluster)  [unwired: 4 in, 7 out]
                  n153 = call "convert_strings.vi"("Enum"=conver_strings_types."RingCMD", "error in (no error)"=w515, "BD Ring Text"=w497, "Instrument Command"=w540) -> ("error out"=w464:errorcluster, "Ring CMD/Enable String"=w462:string)  [unwired: 6 out]
                  n154 = Unbundle By Name(w521) -> ("Left"=w465:u32)
                  n155 = call "cal_multilines_heights_and_widths.vi"("Ring Command"=w462, "Strings And Values []"=w533, "error in (no error)"=w464) -> ("BD Width"=w473:i32, "BD Height"=w475:i32, "error out"=w461:errorcluster)  [unwired: 3 in, 7 out]
                  n156 = Add(x=20, y=w473) -> (x+y=w470:i32)
                  n157 = Add(x=20 ("y"), y=w475) -> (x+y=w474:i32)
                  n158 = call "adjust_position.vi"("Y Offset"=w474, "X Offset"=w465, "Position In"=w513) -> ("Position Out"=w509:cluster{"Left":i32, "Top":i32})  [unwired: 8 out]
                  n159 = Unbundle By Name(w513) -> ("Top"=w468:i32)
                  n160 = Unbundle By Name(w528) -> ("Left"=w517:i32)
                  n161 = Unbundle By Name(w509) -> ("Left"=w471:i32)
                  n162 = Add(x=10, y=w468) -> (x+y=w466:i32)
                  n163 = call "add_percentage_for_floating_datatype.vi"("error in (no error)"=w461, "String In"=w462) -> ("error out"=w498:errorcluster, "String Out"=w499:string)  [unwired: 8 out]
                  n164 = Subtract(x=w471, y=w470) -> (x-y=w469:i32)
                  n165 = Bundle(w469, w466) -> (w524:cluster{i32, i32})  [unwired: 1 out]
                  n166 = call "add_string_constant.vi"("error in"=w498, "BD Position"=w524, "StringConstantValue"=w499, "VI Ref In"=w532) -> ("error out"=w500:errorcluster, "StrCnst Refnum"=w531:refnum<vi>, "VI Ref Out"=w506:refnum<vi>)  [unwired: 5 out]
                  n167 = property class="StrCnst"(reference=w531, error in=w500) -> (reference out=w519:refnum<vi>, error out=w518:errorcluster, "Terminal"=w525:refnum<vi>, "Height"=w530:u32, "Terminal.Top"=w529:i32)
                  n168 = call "find_existing_controls.vi"("error in (no error)"=w500, "Label Text"=w534, "VI Ref In"=w506) -> ("error out"=w503:errorcluster, "New Ctrl"=w505:bool, "Ctrl Ref Out"=w504:refnum<vi>, "VI Ref Out"=w502:refnum<vi>)  [unwired: 5 out]
                  n169 = Compound Arithmetic op=ADD(w530, w529, 10 ("value")) -> (w512:u32)
                  n170 = case shown="True" w505 {
                    tunnel: [w542 w553] -> w527
                    tunnel: [w543 w552] -> w526
                    tunnel: w517 -> [_ w550]
                    tunnel: w535 -> [_ w549]
                    tunnel: w512 -> [_ w547]
                    tunnel: w504 -> [w543 _]
                    tunnel: w503 -> [w542 w546]
                    tunnel: w502 -> [w541 w545]
                    tunnel: [w541 w544] -> w501
                    frame False {
                    }
                    frame True {
                      n171 = Bundle("Left"=w550, w547) -> (w551:cluster{"Left":i32, u32})  [unwired: 1 out]
                      n172 = call "add_control.vi"("Add Control Type"=bd_control_type."Ring" ("Enum"), "error in (no error)"=w546, "Single Control Spec"=w549, "BD Position"=w551, "VI Ref In"=w545) -> ("error out"=w553:errorcluster, "Control Ref Out"=w552:refnum<vi>, "VI Ref Out"=w544:refnum<vi>)  [unwired: 4 out]
                    }
                  }
                  n173 = Subtract(x=w512, y=u32 18) -> (x-y=w510:u32)
                  n174 = Close Reference(reference=w519, error in (no error)=w518) -> (error out=w516:errorcluster)
                  n175 = Bundle By Name(cluster=w509, "Top"=w510) -> (w508:cluster{"Left":i32, "Top":i32})
                  n176 = call "add_node.vi"("Node Type"=node_types."PickLine", "error in (no error)"=w516, "BD Position"=w508, "VI Ref In"=w501) -> ("error out"=w479:errorcluster, "Node Refnum"=w480:refnum<vi>, "VI Ref Out"=w536:refnum<vi>)  [unwired: 2 in, 3 out]
                  n177 = property class="Ctl"(reference=w526, error in=w527) -> (reference out=w495:refnum<vi>, error out=w494:errorcluster, "Terminal"=w491:refnum<vi>)
                  n178 = property class="Node"(reference=w480, error in=w479) -> (reference out=w496:refnum<vi>, error out=w482:errorcluster, "Terms[]"=w493:refnum<vi>[])
                  n179 = Close Reference(reference=w495, error in (no error)=w494) -> (error out=w485:errorcluster)
                  n180 = call "get_string_node_terms.vi"("Terms[] In"=w493, "Node Type"=string_node_type."PickLine", "error in (no error)"=w482) -> ("Terms[]  Out"=w489:refnum<vi>[], "Pick Term"=w490:refnum<vi>, "Multiline Term/Enable Term/Concantenate Term"=w492:refnum<vi>, "error out"=w481:errorcluster)  [unwired: 1 in, 8 out]
                  n181 = Close Reference(reference=w496, error in (no error)=w481) -> (error out=w486:errorcluster)
                  n182 = call "connect_two_terminal.vi"("error in"=w485, "Terminal 2"=w492, "Terminal 1"=w525) -> ("error out"=w487:errorcluster)  [unwired: 1 in, 7 out]
                  n183 = call "connect_two_terminal.vi"("error in"=w487, "Terminal 2"=w491, "Terminal 1"=w490) -> ("error out"=w483:errorcluster)  [unwired: 1 in, 7 out]
                  n184 = call "connect_with_last_node_term.vi"("Last StrCnst Refnum"=w507, "error in (no error)"=w486, "Terminal Index"=w488, "Terminals[]"=w489, "Last Function Ref In"=w523) -> ("error out"=w484:errorcluster)  [unwired: 6 out]
                  n185 = Merge Errors(w484, w483) -> (w537:errorcluster)
                }
              }
            }
          }
        }
      }
    }
    frame Error {
    }
  }
  "error out" <- w6
  "VI Ref Out" <- w4
